vi "connectToDevice.vi"(8 "error in (no error)":errorcluster, 9 "device type (any)":T1 items=["any"=0, "AB1002"=1002, "AB1004"=1004]) -> (0 "error out":errorcluster, 1 "selected device type":T1 items=["any"=0, "AB1002"=1002, "AB1004"=1004], 2 "selected VISA":refnum<visa-resource-name>, 3 "Cancelled?":bool)   [LabVIEW 2015]
doc: "Dialog box\nScans ports for available Tausand Abacus devices, and asks the user to select a device to connect."
uses:
  <instrlib>/Tausand AB1000/Public/Controls/deviceTypeRing.ctl
  <instrlib>/Tausand AB1000/Tausand AB1000.lvlib
panel:
  in  "refresh":bool
  in  "device selector":string(combo)
  out "status":string
  in  "Cancel":bool
  in  "OK":bool
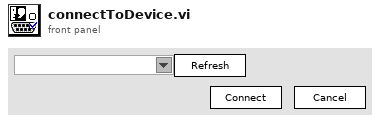
[diagram p1: front panel]
types:
  T1 = typedef "Tausand AB1000.lvlib/deviceTypeRing.ctl" = u16
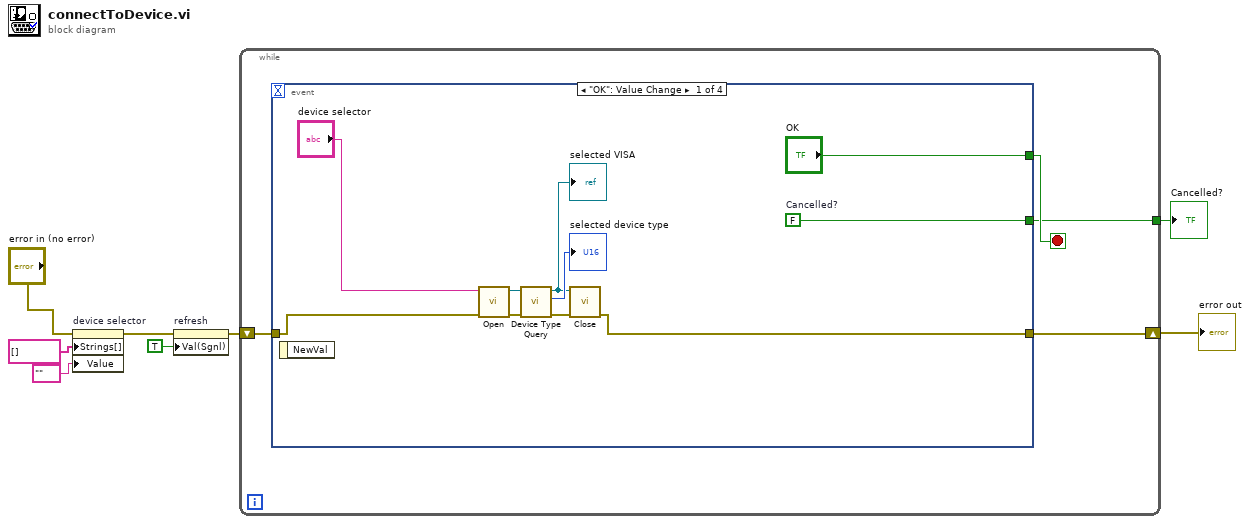
[diagram p0: block diagram]
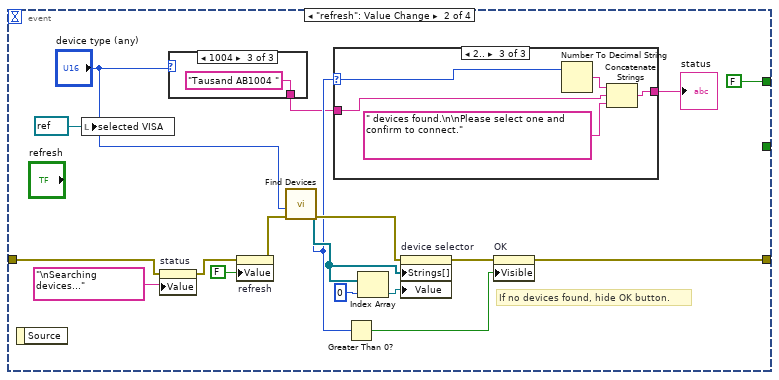
[diagram p2: hidden frame]
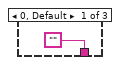
[diagram p3: hidden frame]
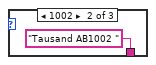
[diagram p4: hidden frame]
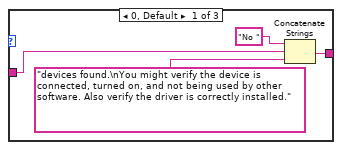
[diagram p5: hidden frame]
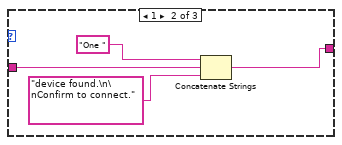
[diagram p6: hidden frame]
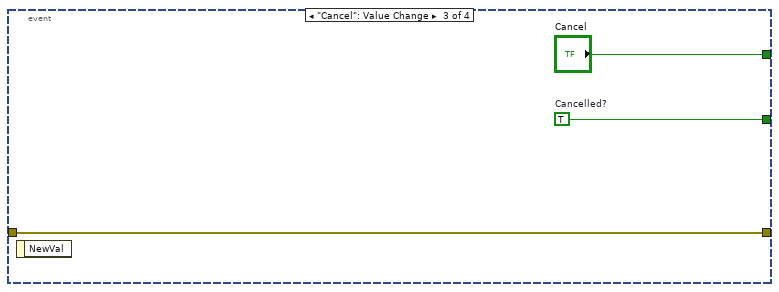
[diagram p7: hidden frame]
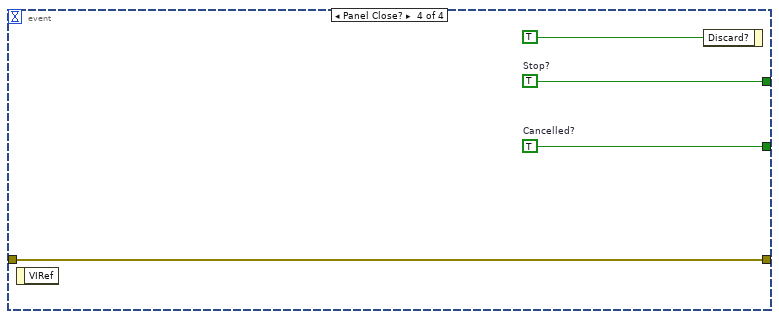
[diagram p8: hidden frame]
diagram:
  n1 = property on="device selector" class="CmbBox"(error in="error in (no error)", "Strings[]"=string[] [] ("Strings []"), "Value"="" ("device selector")) -> (error out=w2:errorcluster)  [unwired: 1 in, 1 out]
  n2 = property on="refresh" class="Bool (strict)"(error in=w2, "Val(Sgnl)"=TRUE) -> (error out=w7:errorcluster)  [unwired: 1 in, 1 out]
  n3 = while {
    tunnel: [w11] -> w8
    shift-right: [w9] -> w5
    shift-left: w7 -> [w10]
    stop <- w12 stop-if-true
    n4 = event shown="[0] \"OK\": Value Change" {
      selector: _ -> [_ _ _ _]
      dyn-events: _ -> [_ _ _ _]
      timeout: _ -> [_ _ _ _]
      tunnel: ["OK" FALSE ("Stop?") "Cancel" w62] -> w12
      tunnel: [w22 _ w59 w61] -> w11
      tunnel: w10 -> [w16 w26 w57 w60]
      tunnel: [w15 w28 w57 w60] -> w9
      event "OK": Value Change {
        w22 = FALSE  # Cancelled?
        n5 = event-data() -> ()  [unwired: 1 in, 1 out]
        n6 = call <instrlib>:"Open.vi"("error in (no error)"=w16, "VISA resource name"="device selector") -> ("error out"=w19:errorcluster, "VISA resource name out"=w13:refnum<visa-resource-name>)  [unwired: 8 in]
        n7 = call <instrlib>:"Device Type Query.vi"("error in (no error)"=w19, "VISA Refnum in"=w13) -> ("error out"=w18:errorcluster, "device type"=→"selected device type":T1, "VISA Refnum out"=w17:refnum<visa-resource-name>)  [unwired: 7 in]
        "selected VISA" <- w17
        n8 = call <instrlib>:"Close.vi"("error in (no error)"=w18, "VISA resource name"=w17) -> ("error out"=w15:errorcluster)  [unwired: 9 in]
      }
      event "refresh": Value Change {
        # "If no devices found, hide OK button."
        n9 = event-data() -> ()  [unwired: 1 in, 1 out]
        n10 = local write "selected VISA"(refnum<visa-resource-name> refnum ("VISA out")) -> ()
        n11 = property on="status" class="Str"(error in=w26, "Value"="\nSearching devices..." ("String")) -> (error out=w25:errorcluster)  [unwired: 1 in, 1 out]
        n12 = case shown="1004" "device type (any)" {
          tunnel: ["" "Tausand AB1002 " ("String") "Tausand AB1004 " ("String")] -> w24
          frame 0, Default {
          }
          frame 1002 {
          }
          frame 1004 {
          }
        }
        n13 = property on="refresh" class="Bool (strict)"(error in=w25, "Value"=FALSE ("Value (Signaling)")) -> (error out=w36:errorcluster)  [unwired: 1 in, 1 out]
        n14 = call <instrlib>:"Find Devices.vi"("error in (no error)"=w36, "device type (any)"="device type (any)") -> ("error out"=w39:errorcluster, "Abacus count"=w31:i32, "Abacus VISAs"=w35:refnum<visa-resource-name>[])  [unwired: 7 in]
        n15 = case shown="2.." w31 {
          selector: w31 -> [_ _ w56]
          tunnel: [w47 w48 w54] -> w38
          tunnel: w24 -> [w44 w50 w52]
          frame 0, Default {
            n16 = Concatenate Strings("No " ("String"), w44, "devices found.\nYou might verify the device is connected, turned on, and not being used by other software. Also verify the driver is correctly installed." ("String")) -> (w47:string)
          }
          frame 1 {
            n17 = Concatenate Strings("One " ("String"), w50, "device found.\n\nConfirm to connect." ("String")) -> (w48:string)
          }
          frame 2.. {
            n18 = Number To Decimal String(number=w56) -> (decimal integer string=w55:string)  [unwired: 1 in]
            n19 = Concatenate Strings(w55, w52, " devices found.\n\nPlease select one and confirm to connect." ("String")) -> (w54:string)
          }
        }
        "status" <- w38
        n20 = Greater Than 0?(x=w31) -> (x > 0?=w30:bool)
        n21 = Index Array(array=w35, index=0) -> (element=w33:refnum<visa-resource-name>)
        n22 = property on="device selector" class="CmbBox"(error in=w39, "Strings[]"=w35, "Value"=w33) -> (error out=w29:errorcluster)  [unwired: 1 in, 1 out]
        n23 = property on="OK" class="Bool"(error in=w29, "Visible"=w30) -> (error out=w28:errorcluster)  [unwired: 1 in, 1 out]
      }
      event "Cancel": Value Change {
        w59 = TRUE  # Cancelled?
        n24 = event-data() -> ()  [unwired: 1 in, 1 out]
      }
      event Panel Close? {
        w61 = TRUE  # Cancelled?
        w62 = TRUE  # Stop?
        n25 = event-data() -> ()  [unwired: 1 in, 1 out]
        n26 = event-data("Discard?"=TRUE) -> ()  [unwired: 1 in, 1 out]
      }
    }
  }
  "Cancelled?" <- w8
  "error out" <- w5
